vi "TDC_configureSignalConditioning.vi"(7 "Edge":i32(ring)=1 items=["Falling", "Rising"], 8 "Error In":errorcluster, 9 "Threshold":dbl format="%#_4pV", 10 "Preset":i32(ring)=1 items=["LVTTL"=1, "NIM"=2, "Misc"=3, "None"=4], 11 "Channel":i32) -> (0 "Error Out":errorcluster)   [LabVIEW 2011]
uses:
  tdcbase.dll
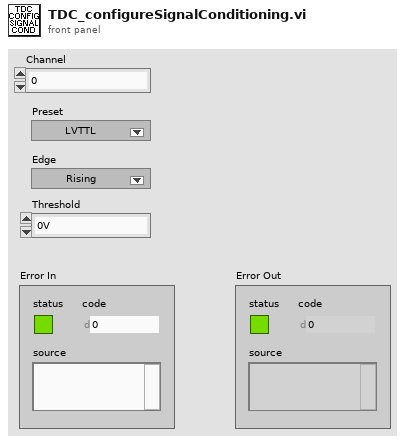
[diagram p1: front panel]
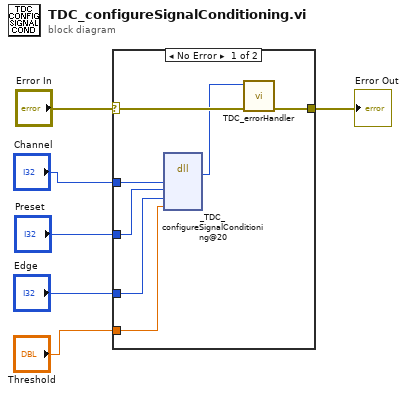
[diagram p0: block diagram]
diagram:
  n1 = case shown="No Error" "Error In" {
    selector: "Error In" -> [w13 w14]
    tunnel: [w12 w14] -> w5
    tunnel: "Channel" -> [w10 _]
    tunnel: "Preset" -> [w9 _]
    tunnel: "Edge" -> [w8 _]
    tunnel: "Threshold" -> [w7 _]
    frame No Error {
      n2 = dll-call lib="X:/tdcbase.dll" fn="_TDC_configureSignalConditioning@20"("channel"=w10, "conditioning"=w9, "edge"=w8, "threshold"=w7) -> ("return type"=w11:i32)  [unwired: 7 in, 2 out]
      n3 = call "TDC_errorHandler.vi"("Error In"=w13, "TDC Return Code"=w11) -> ("Error Out"=w12:errorcluster)  [unwired: 9 in]
    }
    frame Error {
    }
  }
  "Error Out" <- w5
